vi "Get PCM Data.vi"(0 "Pneumatics Control Module (0)":u8, 11 "error in":errorcluster) -> (6 "PCM Data Out":T1, 15 "error out":errorcluster)   [LabVIEW 2014]
doc: "Returns the current of the compressor on the Pneumatics Control Module (PCM)."
uses:
  PCM Data.ctl
  <vilib>/Rock Robotics/WPI/CAN/PCM/WPI_CAN_PCMGlobalOps.ctl
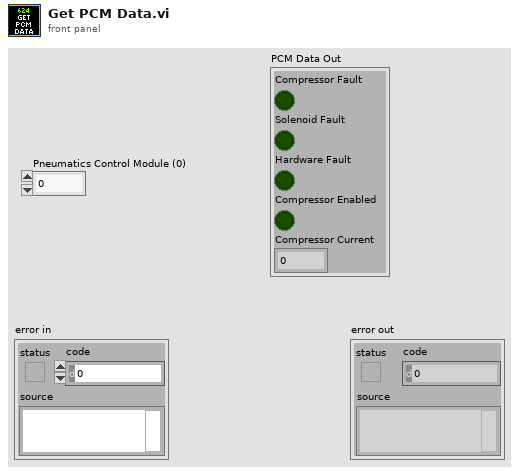
[diagram p1: front panel]
types:
  T1 = typedef "PCM Data.ctl" = cluster{"Compressor Fault":bool, "Solenoid Fault":bool, "Compressor Enabled":bool, "Hardware Fault":bool, "Compressor Current":dbl}
  T2 = typedef "WPI_CAN_PCMGlobalOps.ctl" = enum16{"Read For Send", "Write After Receive", "Set Solenoids", "Set Closed Loop", "Clear Sticky Faults", "Get All", "Write Error", "Write After Receive Blacklist"}
  T3 = cluster{"Solenoid Status":bool[], "Battery Voltage":dbl, "Solenoid Voltage":dbl, "Compressor Current":dbl, "CompressorEnabled":bool, "StickySolenoidFault":bool, "StickyCompressorFault":bool, "SolenoidFault":bool, "CompressorFault":bool, "HardwareFault":bool, "ClosedLoopStatus":bool, "PressureStatus":bool, "Module Enabled":bool, "ClosedLoopSuggestedOutput":bool, "CAN Error":errorcluster, "Sticky Solenoid Faults":bool[]}
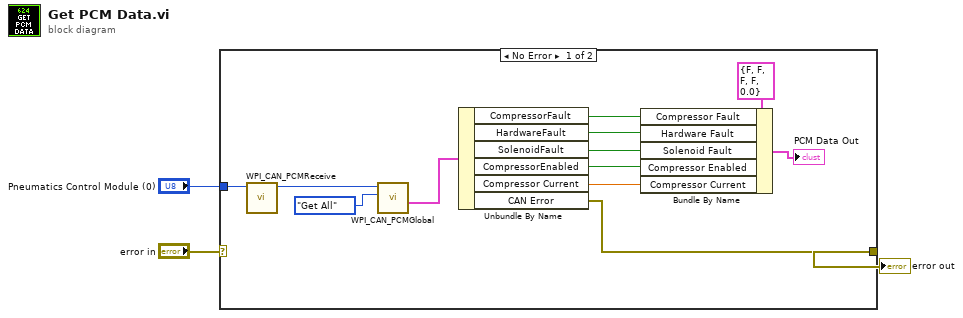
[diagram p0: block diagram]
diagram:
  n1 = case shown="No Error" "error in" {
    selector: "error in" -> [_ w16]
    tunnel: [w11 w16] -> w2
    tunnel: "Pneumatics Control Module (0)" -> [w12 _]
    frame No Error {
      n2 = call <vilib>:"WPI_CAN_PCMReceive.vi"("Pneumatics Control Module (0)"=w12) -> ("Pneumatics Control Module Out"=w14:u8)  [unwired: 10 in]
      n3 = call <vilib>:"WPI_CAN_PCMGlobal.vi"("Operation"=WPI_CAN_PCMGlobalOps."Get All", "Pneumatics Control Module (0)"=w14) -> ("Get All"=w15:T3)  [unwired: 7 in, 2 out]
      n4 = Unbundle By Name(w15) -> ("CompressorFault"=w5:bool, "HardwareFault"=w6:bool, "SolenoidFault"=w7:bool, "CompressorEnabled"=w8:bool, "Compressor Current"=w9:dbl, "CAN Error"=w11:errorcluster)
      n5 = Bundle By Name(cluster=T1 {"Compressor Fault"=FALSE, "Solenoid Fault"=FALSE, "Compressor Enabled"=FALSE, "Hardware Fault"=FALSE, "Compressor Current"=0.0} ("input cluster"), "Compressor Fault"=w5, "Hardware Fault"=w6, "Solenoid Fault"=w7, "Compressor Enabled"=w8, "Compressor Current"=w9) -> (→"PCM Data Out":T1)
    }
    frame Error {
    }
  }
  "error out" <- w2
